vi "MCL Ramping.vi"(3 "error in (no error)":errorcluster, 4 "timeout":i32=200, 6 "MCL State In":refnum<queue>) -> (0 "error out":errorcluster, 1 "Is Ramping?":bool, 2 "MCL State Out":refnum<queue>)   [LabVIEW 2013]
uses:
  MixedMode/MCL States.ctl
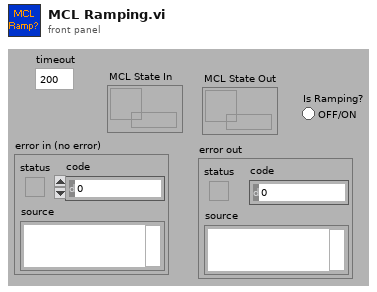
[diagram p1: front panel]
types:
  T1 = typedef "MCL States.ctl" = enum16{"MCL Idle", "MCL Ramping", "MCL Holding", "MCL Aborting", "MCL Done", "MCL NOP"}
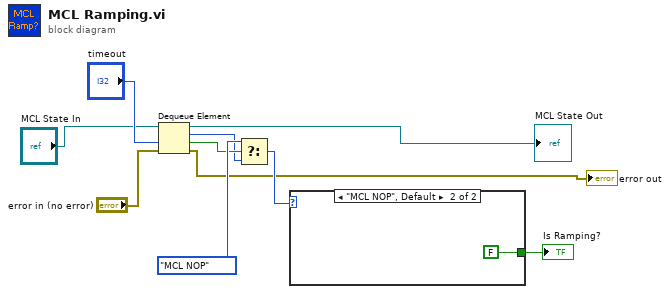
[diagram p0: block diagram]
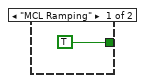
[diagram p2: hidden frame]
diagram:
  n1 = Dequeue Element(queue="MCL State In", timeout in ms (-1)="timeout", error in (no error)="error in (no error)") -> (queue out=→"MCL State Out":refnum<queue>, element=w4:T1, timed out?=w9:bool, error out=→"error out":errorcluster)
  n2 = Select(t=MCL_States."MCL NOP", s=w9, f=w4) -> (s? t:f=w8:T1)
  n3 = case shown="\"MCL NOP\", Default" w8 {
    tunnel: [TRUE FALSE] -> w1
    frame "MCL Ramping" {
    }
    frame "MCL NOP", Default {
    }
  }
  "Is Ramping?" <- w1
